vi "AD7609_Sample9606.vi"() -> (0 "OK":bool, 1 "FRSTDATA":bool[](array[boolean]), 3 "DATA":i16[](array[numeric])=[9827, -1, 0, -1, -1, 1, 3, 13138])   [LabVIEW 2012]
uses:
  glADC.vi
  <vilib>/rvi/eio/common/nirviEmuTemplateMethod_errors.vi
  <vilib>/eio/EIONode/EIONode.xnode
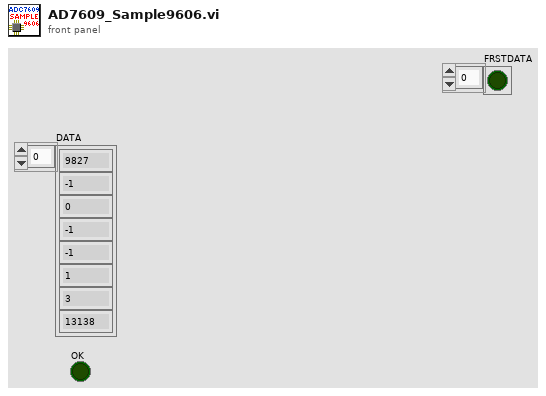
[diagram p1: front panel]
types:
  T1 = cluster{"OS":u8, "Range":u8, "T_hi":u8, "D_low":u8}
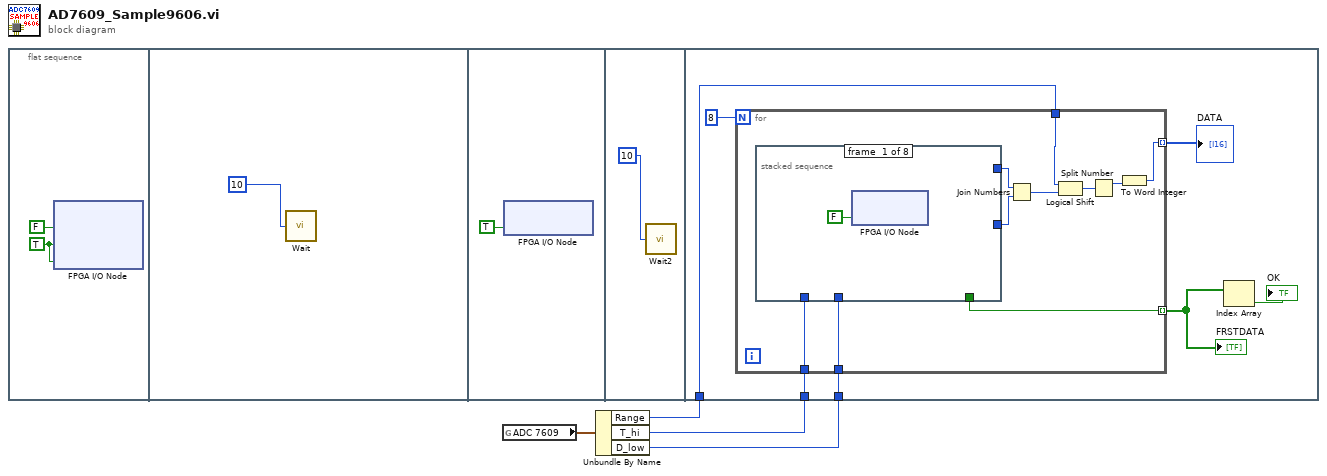
[diagram p0: block diagram]
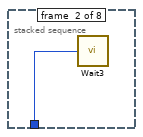
[diagram p2: hidden frame]
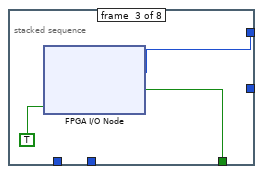
[diagram p3: hidden frame]
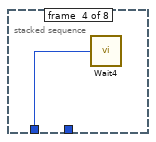
[diagram p4: hidden frame]
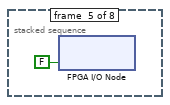
[diagram p5: hidden frame]
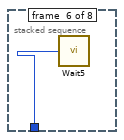
[diagram p6: hidden frame]
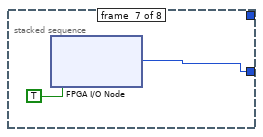
[diagram p7: hidden frame]
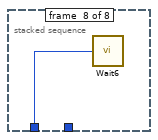
[diagram p8: hidden frame]
diagram:
  n1 = flat-sequence {
    tunnel: w1 -> [w15]
    tunnel: w2 -> [w14]
    tunnel: w3 -> [w10]
    frame #0 {
      w5 = TRUE ("RD2")
      n2 = xnode "FPGA I/O Node"("CONVST1"=FALSE ("RESET"), "RD2"=w5, "CONVST2"=w5) -> ()  [unwired: 3 in, 3 out]
    }
    frame #1 {
      n3 = call "Wait"("Count(Ticks)"=u8 10 ("T_convst")) -> ()  [unwired: 1 out]
    }
    frame #2 {
      n4 = xnode "FPGA I/O Node"("CONVST1"=TRUE ("RESET")) -> ()  [unwired: 1 in, 1 out]
    }
    frame #3 {
      n5 = call "Wait2"("Count(Ticks)"=u8 10 ("D_convst")) -> ()  [unwired: 1 out]
    }
    frame #4 {
      n6 = for {
        N: 8 -> [_]
        tunnel: [w18] -> w13 mode=indexing
        tunnel: [w26] -> w11 mode=indexing
        tunnel: w15 -> [w25]
        tunnel: w14 -> [w24]
        tunnel: w10 -> [w17]
        n7 = stacked-sequence {
          tunnel: [_ _ w29 _ _ _ _ _] -> w23
          tunnel: [_ _ w31 _ _ _ _ _] -> w26
          tunnel: [_ _ _ _ _ _ w35 _] -> w22
          tunnel: w25 -> [_ w28 _ _ _ w34 _ _]
          tunnel: w24 -> [_ _ _ w32 _ _ _ w37]
          frame #0 {
            n8 = xnode "FPGA I/O Node"("RD1"=FALSE ("RD")) -> ()  [unwired: 1 in, 1 out]
          }
          frame #1 {
            n9 = call "Wait3"("Count(Ticks)"=w28) -> ()  [unwired: 1 out]
          }
          frame #2 {
            n10 = xnode "FPGA I/O Node"("RD1"=TRUE ("RD")) -> ("DB0-DB15"=w29:u16, "FRSTDATA1"=w31:bool)  [unwired: 3 in, 3 out]
          }
          frame #3 {
            n11 = call "Wait4"("Count(Ticks)"=w32) -> ()  [unwired: 1 out]
          }
          frame #4 {
            n12 = xnode "FPGA I/O Node"("RD1"=FALSE ("RESET")) -> ()  [unwired: 1 in, 1 out]
          }
          frame #5 {
            n13 = call "Wait5"("Count(Ticks)"=w34) -> ()  [unwired: 1 out]
          }
          frame #6 {
            n14 = xnode "FPGA I/O Node"("RD1"=TRUE ("RD")) -> ("DB0-DB15"=w35:u16)  [unwired: 2 in, 2 out]
          }
          frame #7 {
            n15 = call "Wait6"("Count(Ticks)"=w37) -> ()  [unwired: 1 out]
          }
        }
        n16 = Join Numbers(hi=w23, lo=w22) -> ((hi.lo)=w21:u32)
        n17 = Logical Shift(y=w17, x=w21) -> (x << y=w20:u32)
        n18 = Split Number(x=w20) -> (hi(x)=w19:u16)  [unwired: 1 out]
        n19 = To Word Integer(number=w19) -> (16bit integer=w18:i16)
      }
      "DATA" <- w13
      "FRSTDATA" <- w11
      n20 = Index Array(array=w11) -> (element=→"OK":bool)  [unwired: 1 in]
    }
  }
  n21 = global read "glADC.vi" "ADC 7609"() -> (w4:T1)
  n22 = Unbundle By Name(w4) -> ("Range"=w3:u8, "T_hi"=w2:u8, "D_low"=w1:u8)
